vi "CRYSet Multimeter Front Panel.vi"(11 "Vi Ref in":refnum<vi> caption="Vi Ref") -> (3 "Vi Ref out":refnum<vi> caption="Vi Ref")   [LabVIEW 2013]
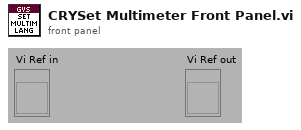
[diagram p1: front panel]
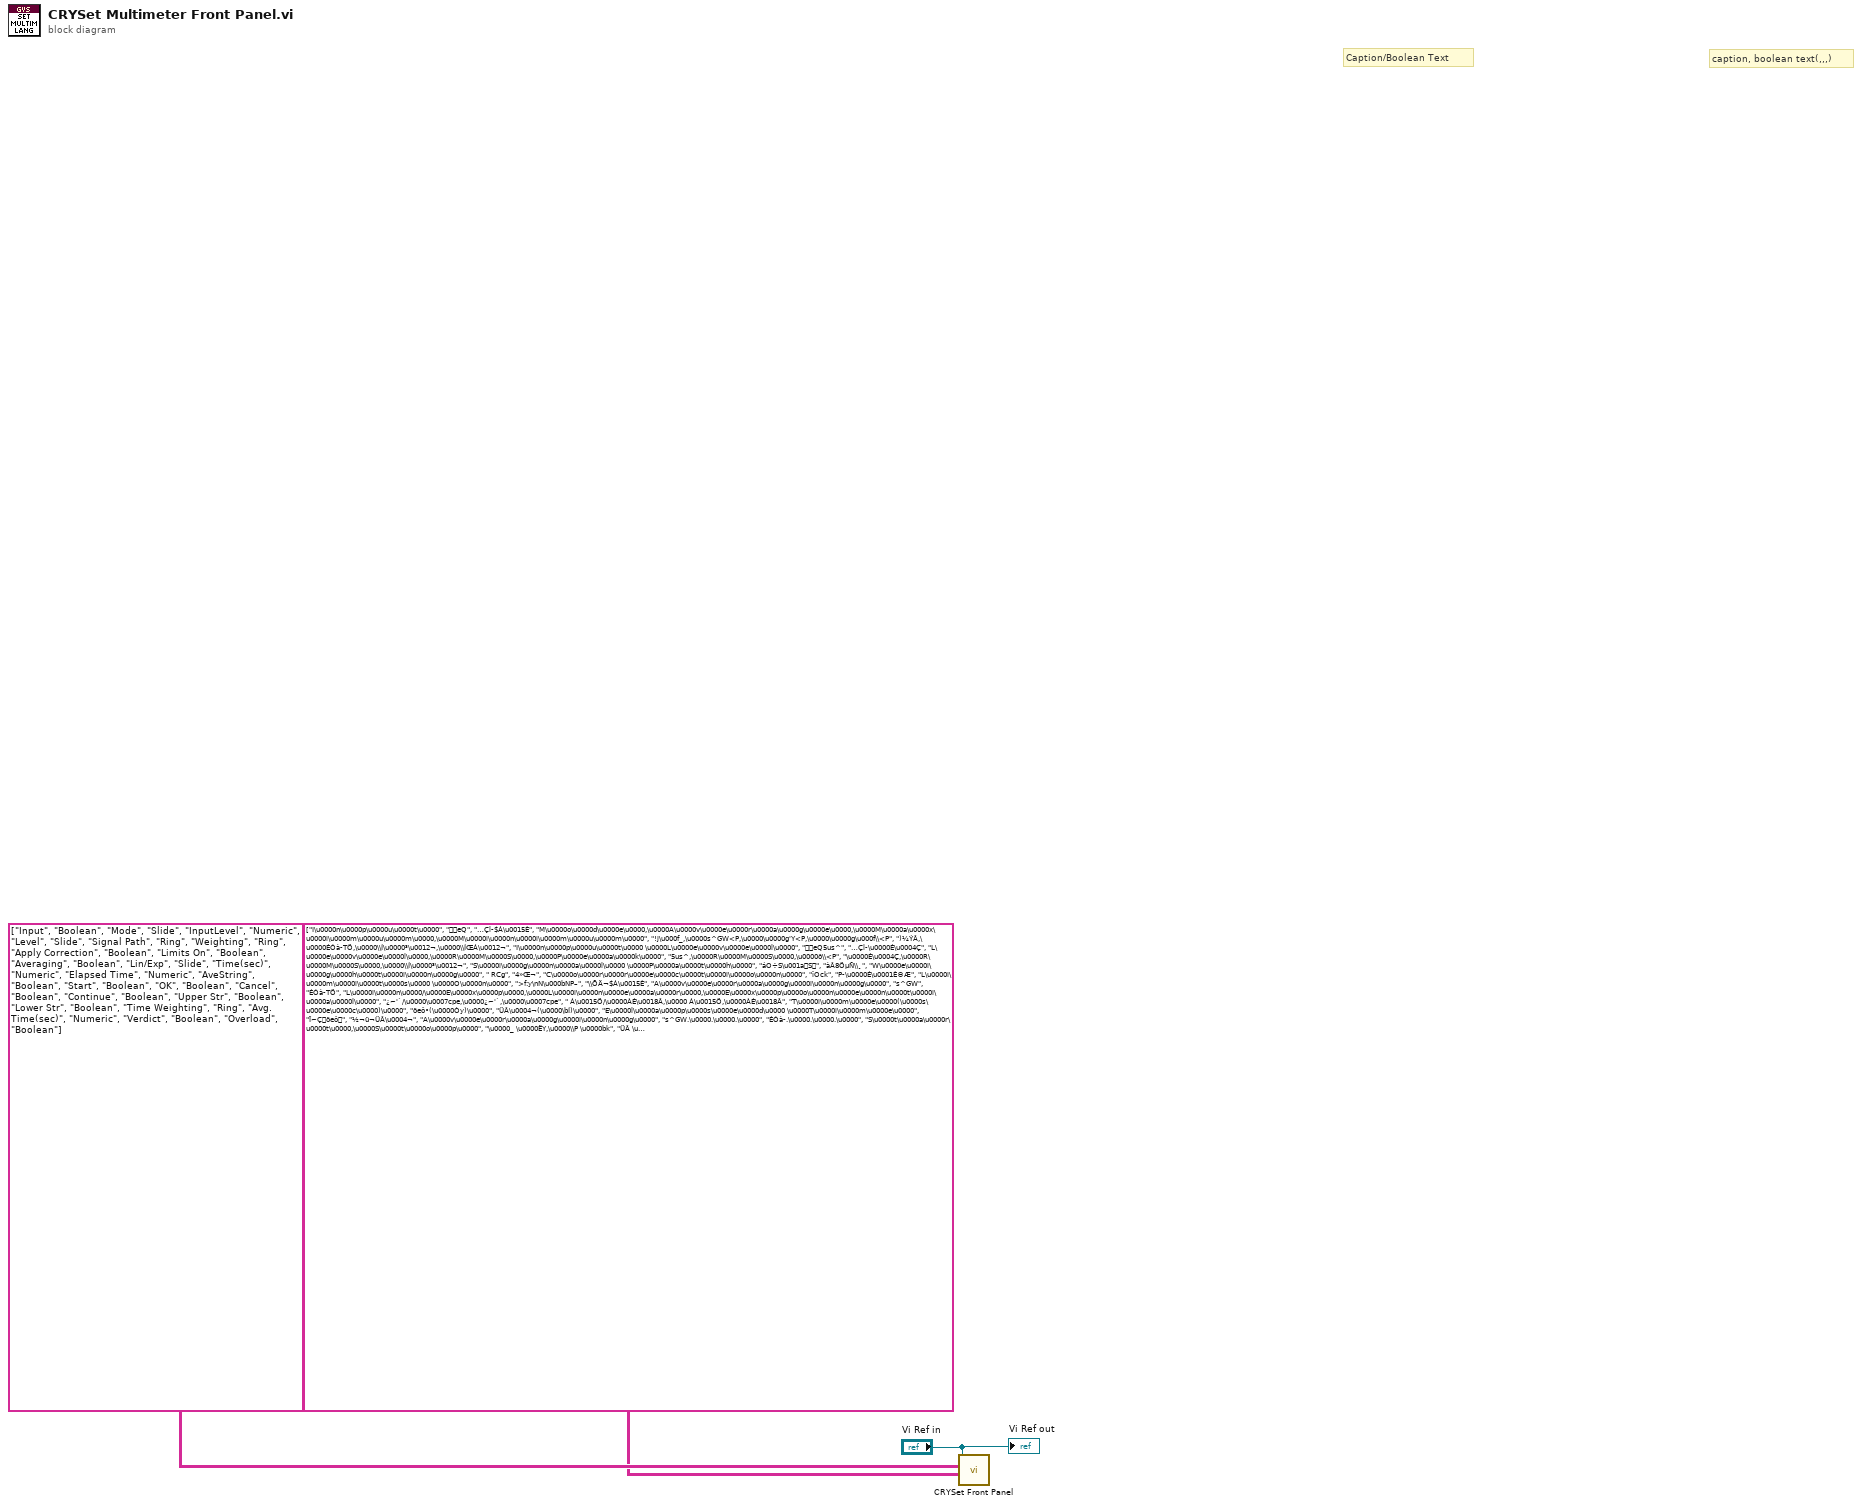
[diagram p0: block diagram]
diagram:
  # "caption, boolean text(,,,)"
  # "Caption/Boolean Text"
  n1 = call "CRYSet Front Panel.vi"("Caption(Boolean Text)"=string[][] [["I\u0000n\u0000p\u0000u\u0000t\u0000", "eQ", "…Çl­$Á\u0015È"], ["M\u0000o\u0000d\u0000e\u0000,\u0000A\u0000v\u0000e\u0000r\u0000a\u0000g\u0000e\u0000,\u0000M\u0000a\u0000x\u0000i\u0000m\u0000u\u0000m\u0000,\u0000M\u0000i\u0000n\u0000i\u0000m\u0000u\u0000m\u0000", "!j\u000f_,\u0000s^GW<P,\u0000\u0000g'Y<P,\u0000\u0000g\u000f\\<P", ")¼ÝÂ,\u0000ÉÓà­TÖ,\u0000\\Í\u0000³\u0012¬,\u0000\\ÍŒÁ\u0012¬"], ["I\u0000n\u0000p\u0000u\u0000t\u0000 \u0000L\u0000e\u0000v\u0000e\u0000l\u0000", "eQ5us^", "…Çl­\u0000É\u0004Ç"], ["L\u0000e\u0000v\u0000e\u0000l\u0000,\u0000R\u0000M\u0000S\u0000,\u0000P\u0000e\u0000a\u0000k\u0000", "5us^,\u0000R\u0000M\u0000S\u0000,\u0000ð\\<P", "\u0000É\u0004Ç,\u0000R\u0000M\u0000S\u0000,\u0000\\Í\u0000³\u0012¬"], ["S\u0000i\u0000g\u0000n\u0000a\u0000l\u0000 \u0000P\u0000a\u0000t\u0000h\u0000", "áO÷S\u001aS", "àÂ8ÖµÑ\\¸"], ["W\u0000e\u0000i\u0000g\u0000h\u0000t\u0000i\u0000n\u0000g\u0000", " RCg", "4»Œ¬"], ["C\u0000o\u0000r\u0000r\u0000e\u0000c\u0000t\u0000i\u0000o\u0000n\u0000", "îOck", "P­\u0000É\u0001È©Æ"], ["L\u0000i\u0000m\u0000i\u0000t\u0000s\u0000 \u0000O\u0000n\u0000", ">f:y\nN\u000bNP–", "\\ÕÄ¬$Á\u0015È"], ["A\u0000v\u0000e\u0000r\u0000a\u0000g\u0000i\u0000n\u0000g\u0000", "s^GW", "ÉÓà­TÖ"], ["L\u0000i\u0000n\u0000/\u0000E\u0000x\u0000p\u0000,\u0000L\u0000i\u0000n\u0000e\u0000a\u0000r\u0000,\u0000E\u0000x\u0000p\u0000o\u0000n\u0000e\u0000n\u0000t\u0000i\u0000a\u0000l\u0000", "¿~'`/\u0000\u0007cpe,\u0000¿~'`,\u0000\u0007cpe", " Á\u0015Ö/\u0000ÀÉ\u0018Â,\u0000 Á\u0015Ö,\u0000ÀÉ\u0018Â"], ["T\u0000i\u0000m\u0000e\u0000(\u0000s\u0000e\u0000c\u0000)\u0000", "öeô•(\u0000Òy)\u0000", "ÜÂ\u0004¬(\u0000\bÍ)\u0000"], ["E\u0000l\u0000a\u0000p\u0000s\u0000e\u0000d\u0000 \u0000T\u0000i\u0000m\u0000e\u0000", "Ï~Çöeô", "½¬ü¬ÜÂ\u0004¬"], ["A\u0000v\u0000e\u0000r\u0000a\u0000g\u0000i\u0000n\u0000g\u0000", "s^GW.\u0000.\u0000.\u0000", "ÉÓà­.\u0000.\u0000.\u0000"], ["S\u0000t\u0000a\u0000r\u0000t\u0000,\u0000S\u0000t\u0000o\u0000p\u0000", "\u0000_ \u0000ËY,\u0000\\P \u0000bk", "ÜÂ \u0000‘Ç,\u0000\u0015È \u0000ÀÉ"], ["O\u0000K\u0000", "nx¤‹", "UÖxÇ"], ["C\u0000a\u0000n\u0000c\u0000e\u0000l\u0000", "ÖSˆm", "èÍŒÁ"], ["C\u0000o\u0000n\u0000t\u0000i\u0000n\u0000u\u0000e\u0000", "Þí~", "Ä¬ \u0000Á"], ["U\u0000p\u0000p\u0000e\u0000r\u0000 \u0000l\u0000i\u0000m\u0000i\u0000t\u0000,\u0000U\u0000p\u0000p\u0000e\u0000r\u0000 \u0000l\u0000i\u0000m\u0000i\u0000t\u0000", "\nNP–,\u0000\nNP–", "ÃÆ\\ÕÄ¬,\u0000ÃÆ\\ÕÄ¬"], ["L\u0000o\u0000w\u0000e\u0000r\u0000 \u0000l\u0000i\u0000m\u0000i\u0000t\u0000,\u0000L\u0000o\u0000w\u0000e\u0000r\u0000 \u0000l\u0000i\u0000m\u0000i\u0000t\u0000", "\u000bNP–,\u0000\u000bNP–", "DÅ˜·\\ÕÄ¬,\u0000DÅ˜·\\ÕÄ¬"], ["T\u0000i\u0000m\u0000e\u0000 \u0000W\u0000e\u0000i\u0000g\u0000h\u0000t\u0000", "öeô•¡‹Cg", "ÜÂ\u0004¬4»Œ¬TÖ"], ["A\u0000v\u0000g\u0000.\u0000T\u0000i\u0000m\u0000e\u0000(\u0000s\u0000e\u0000c\u0000)\u0000", "s^GWöeô•(\u0000Òy)\u0000", "ÜÂ\u0004¬ÉÓà­(\u0000\bÍ)\u0000"], ["F\u0000a\u0000i\u0000l\u0000e\u0000d\u0000,\u0000P\u0000a\u0000s\u0000s\u0000e\u0000d\u0000", "1Y%,\u0000\u001aÇ", "ˆ½µÑü¬,\u0000µÑü¬"], ["O\u0000V\u0000E\u0000R\u0000L\u0000O\u0000A\u0000D\u0000", "Ç \u0000 \u0000}", "\\ÕÄ¬\u0018±hÎ"]], "Control ID and Type(Label Name, Type)"=string[][] [["Input", "Boolean"], ["Mode", "Slide"], ["InputLevel", "Numeric"], ["Level", "Slide"], ["Signal Path", "Ring"], ["Weighting", "Ring"], ["Apply Correction", "Boolean"], ["Limits On", "Boolean"], ["Averaging", "Boolean"], ["Lin/Exp", "Slide"], ["Time(sec)", "Numeric"], ["Elapsed Time", "Numeric"], ["AveString", "Boolean"], ["Start", "Boolean"], ["OK", "Boolean"], ["Cancel", "Boolean"], ["Continue", "Boolean"], ["Upper Str", "Boolean"], ["Lower Str", "Boolean"], ["Time Weighting", "Ring"], ["Avg.Time(sec)", "Numeric"], ["Verdict", "Boolean"], ["Overload", "Boolean"]], "Vi Ref"="Vi Ref in") -> ()  [unwired: 9 in]
  "Vi Ref out" <- "Vi Ref in"
